vi "Configure Active Compliance.vi"(8 "error in (no error)":errorcluster, 9 "Active Compliance Settings":T1={"Clockwise Slope (9.38416 deg)"=9.384164, "Counter-Clockwise Slope (9.38416 deg)"=9.384164, "Clockwise Margin (0.293255 deg)"=0.29325512, "Counter-Clockwise Margin (0.293255 deg)"=0.29325512, "Punch (3.12805%)"=3.12805, "Max  Torque (100%)"=100.0}, 10 "Motor ID (0)":u8, 11 "Dynamixel Motor VISA in":refnum<class "Dynamixel Motor VISA.lvclass">) -> (0 "error out":errorcluster, 3 "Dynamixel Motor VISA out":refnum<class "Dynamixel Motor VISA.lvclass">)   [LabVIEW 2016, in "Dynamixel Motor VISA.lvclass"]
doc: "Adjusts the active compliance of the motor. See the motor's user manual for more details."
uses:
  <instrlib>/Dynamixel Motor/HAIOL/VISA/Dynamixel Motor VISA.lvclass
  <instrlib>/Dynamixel Motor/Public/Configure/Active Compliance Settings.ctl
  <instrlib>/Dynamixel Motor/HAIOL/VISA/Dynamixel Motor VISA.lvclass/Dynamixel Motor VISA.ctl
  <instrlib>/Dynamixel Motor/Dynamixel Motor.lvlib
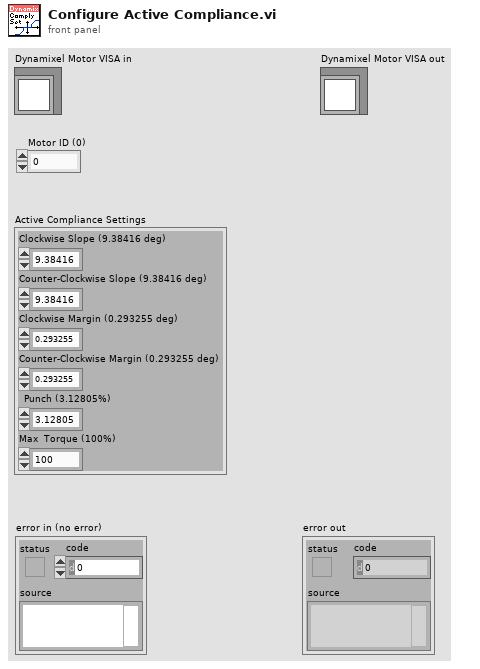
[diagram p1: front panel]
types:
  T1 = typedef "Dynamixel Motor.lvlib/Active Compliance Settings.ctl" = cluster{"Clockwise Slope (9.38416 deg)":sgl, "Counter-Clockwise Slope (9.38416 deg)":sgl, "Clockwise Margin (0.293255 deg)":sgl, "Counter-Clockwise Margin (0.293255 deg)":sgl, "Punch (3.12805%)":sgl, "Max  Torque (100%)":sgl}
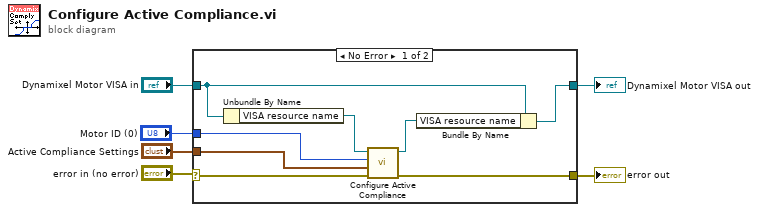
[diagram p0: block diagram]
diagram:
  n1 = case shown="No Error" "error in (no error)" {
    selector: "error in (no error)" -> [w14 w15]
    tunnel: "Dynamixel Motor VISA in" -> [w8 w16]
    tunnel: "Motor ID (0)" -> [w12 _]
    tunnel: "Active Compliance Settings" -> [w11 _]
    tunnel: [w10 w15] -> w2
    tunnel: [w7 w16] -> w1
    frame No Error {
      n2 = Unbundle By Name(w8) -> ("VISA resource name"=w13:refnum<visa-resource-name>)
      n3 = call <instrlib>:"Configure Active Compliance.vi"("error in (no error)"=w14, "Active Compliance Settings"=w11, "Motor ID (0)"=w12, "VISA resource name"=w13) -> ("error out"=w10:errorcluster, "VISA resource name out"=w9:refnum<visa-resource-name>)  [unwired: 6 in]
      n4 = Bundle By Name(cluster=w8, "VISA resource name"=w9) -> (w7:refnum<class "Dynamixel Motor VISA.lvclass">)
    }
    frame Error {
    }
  }
  "error out" <- w2
  "Dynamixel Motor VISA out" <- w1
